vi "Write Test VIs.vi"(8 "error in (no error)":errorcluster, 10 "Test VIs":path[](array[path]), 11 "Test Runner in":refnum<class "Test Runner.lvclass">) -> (0 "error out":errorcluster, 3 "Test Runner out":refnum<class "Test Runner.lvclass">)   [LabVIEW 2013, in "Caraya.lvlib" / "Test Runner.lvclass"]
uses:
  Test Runner.lvclass
  Test Runner.lvclass/Test Runner.ctl
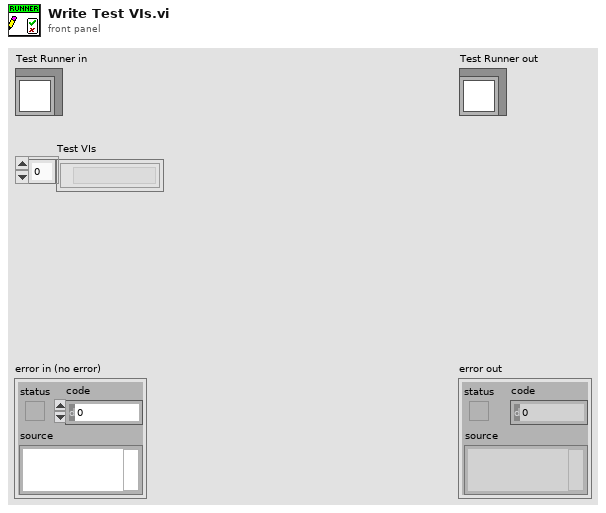
[diagram p1: front panel]
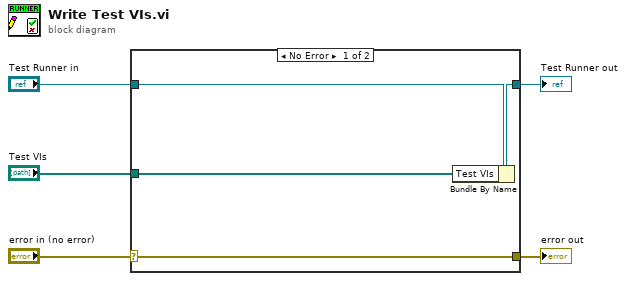
[diagram p0: block diagram]
diagram:
  n1 = case shown="No Error" "error in (no error)" {
    selector: "error in (no error)" -> [w9 w10]
    tunnel: [w9 w10] -> w4
    tunnel: [w7 w11] -> w2
    tunnel: "Test Runner in" -> [w8 w11]
    tunnel: "Test VIs" -> [w6 _]
    frame No Error {
      n2 = Bundle By Name(cluster=w8, "Test VIs"=w6) -> (w7:refnum<class "Test Runner.lvclass">)
    }
    frame Error {
    }
  }
  "error out" <- w4
  "Test Runner out" <- w2
